vi "Clear Log.vi"(8 "error in (no error)":errorcluster, 11 "Normal Log in":refnum<class "Normal Log.lvclass">) -> (0 "error out":errorcluster, 3 "Normal Log out":refnum<class "Normal Log.lvclass">)   [LabVIEW 2020, in "Normal Log.lvlib" / "Normal Log.lvclass"]
uses:
  Normal Log.lvclass
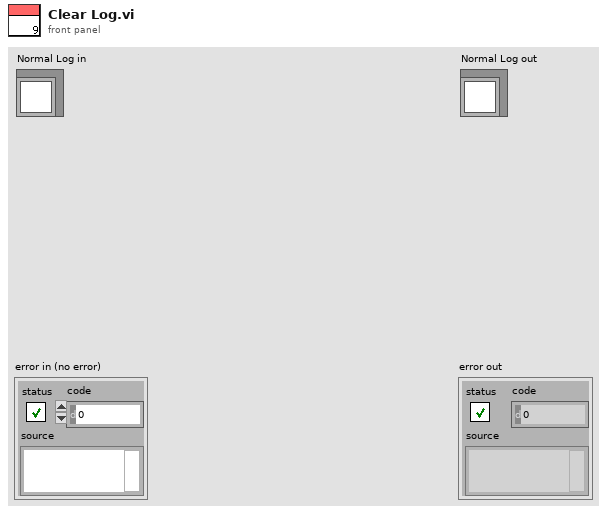
[diagram p1: front panel]
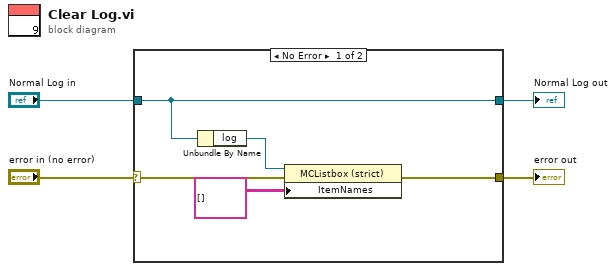
[diagram p0: block diagram]
diagram:
  n1 = case shown="No Error" "error in (no error)" {
    selector: "error in (no error)" -> [w8 w11]
    tunnel: [w5 w11] -> w2
    tunnel: "Normal Log in" -> [w9 w10]
    tunnel: [w9 w10] -> w1
    frame No Error {
      n2 = Unbundle By Name(w9) -> ("log"=w7:refnum<vi>)
      n3 = property class="MCListbox (strict)"(reference=w7, error in=w8, "ItemNames"=string[][] [] ("Item Names")) -> (error out=w5:errorcluster)  [unwired: 1 out]
    }
    frame Error {
    }
  }
  "error out" <- w2
  "Normal Log out" <- w1
